vi "odor config array to odor-color map (sub-vi).vi"(10 "odor config array":T1) -> (2 "odor-color map":T5)   [LabVIEW 2021]
uses:
  type-defs/odor channel to odor color map (type def).ctl
  type-defs/odor selection (type def).ctl
  type-defs/odor color (type def).ctl
  type-defs/odor description array (type def).ctl
  type-defs/odor info cluster (type def).ctl
  type-defs/odor color enum (type def).ctl
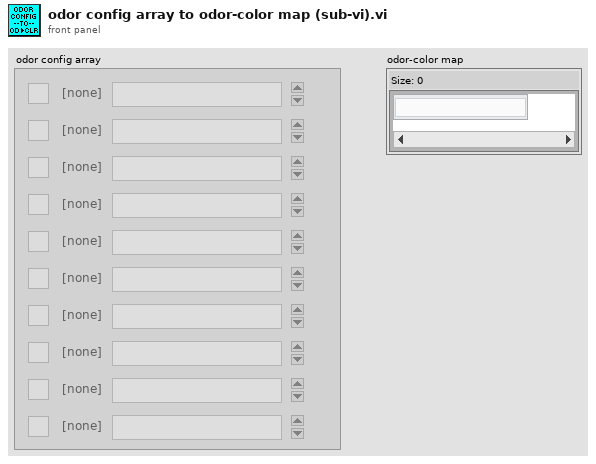
[diagram p1: front panel]
types:
  T1 = typedef "odor description array (type def).ctl" = T2[]
  T2 = typedef "odor info cluster (type def).ctl" = cluster{"odor channel":T3, "odor description":string, "odor color":T4, "odor channel active":bool}
  T3 = typedef "odor selection (type def).ctl" = enum16{"[none]", "odor 1", "odor 2", "odor 3", "odor 4", "odor 5", "odor 6", "odor 7", "odor 8", "odor 9", "odor 10"}
  T4 = typedef "odor color (type def).ctl" = u16
  T5 = typedef "odor channel to odor color map (type def).ctl" = map{T3, T4}
  T6 = typedef "odor color enum (type def).ctl" = enum16{"white", "blue", "red", "orange", "yellow", "green", "magenta", "brown", "black", "[none]"}
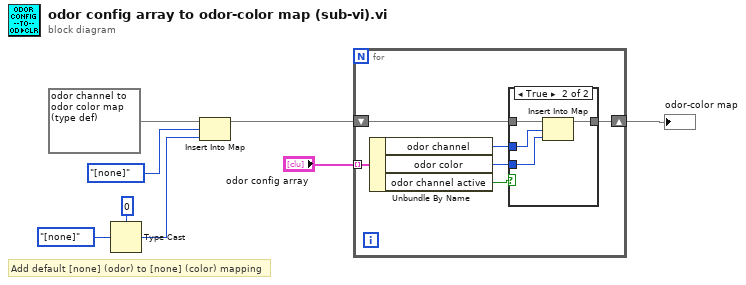
[diagram p0: block diagram]
diagram:
  # "Add default [none] (odor) to [none] (color) mapping"
  n1 = Type Cast(type=T4 0 ("value"), x=odor_color_enum_(type_def)."[none]" ("Enum")) -> (*(type *) &x=w3:T4)
  n2 = Insert Into Map(map in=T5 {}, key=odor_selection_(type_def)."[none]", value=w3) -> (map out=w6:T5)  [unwired: 2 out]
  n3 = for {
    tunnel: "odor config array" -> [w14] mode=indexing
    shift-right: [w10] -> w8
    shift-left: w6 -> [w11]
    n4 = Unbundle By Name(w14) -> ("odor channel"=w13:T3, "odor color"=w12:T4, "odor channel active"=w9:bool)
    n5 = case shown="True" w9 {
      tunnel: w13 -> [_ w19]
      tunnel: w12 -> [_ w18]
      tunnel: w11 -> [w15 w17]
      tunnel: [w15 w16] -> w10
      frame False {
      }
      frame True {
        n6 = Insert Into Map(map in=w17, key=w19, value=w18) -> (map out=w16:T5)  [unwired: 2 out]
      }
    }
  }
  "odor-color map" <- w8
